vi "merge tdms files.vi"(0 "save to":path, 5 "merge paths":path[](array[path])) -> (14 "Dateipfad (Ausgang)":path, 19 "Fehler (Ausgang)":errorcluster)   [LabVIEW 2010, in "util.lvlib"]
uses:
  util.lvlib
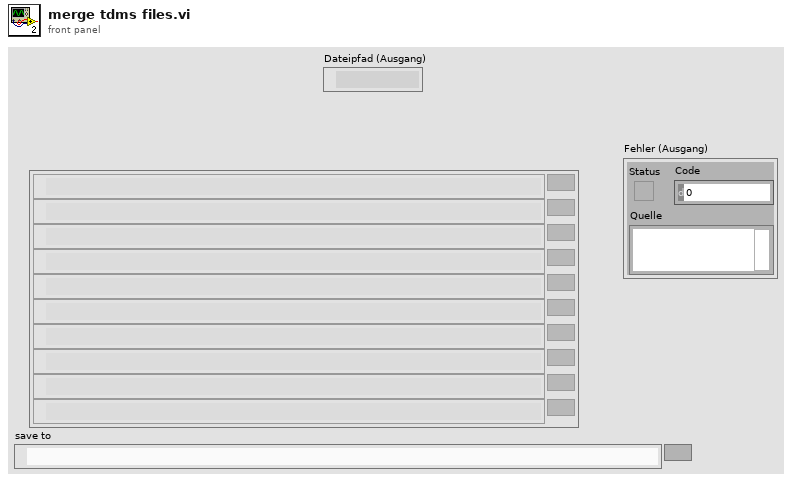
[diagram p1: front panel]
types:
  T1 = enum16{"open", "open or create", "create or replace", "create", "open (read-only)"}
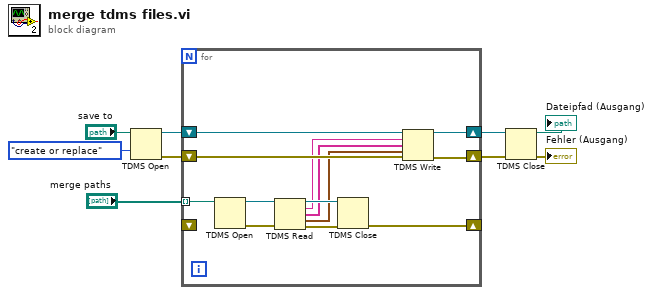
[diagram p0: block diagram]
diagram:
  n1 = TDMS Open(10:T1."create or replace" ("Operation (0:Öffnen)"), 11:"save to") -> (0:w8:errorcluster, 3:w9:refnum<k34>)  [unwired: 4 in]
  n2 = for {
    tunnel: "merge paths" -> [w22] mode=indexing
    shift-right: [w17] -> _
    shift-left: _ -> [_]
    shift-right: [w13] -> w7
    shift-left: w8 -> [w14]
    shift-right: [w15] -> w6
    shift-left: w9 -> [w16]
    n3 = TDMS Open(11:w22) -> (0:w19:errorcluster, 3:w21:refnum<k34>)  [unwired: 5 in]
    n4 = TDMS Read(0:w21, 11:w19) -> (4:w20:refnum<k34>, 6:w12:string, 8:w11:string[], 10:w10:waveform(dbl)[], 15:w18:errorcluster)  [unwired: 5 in, 1 out]
    n5 = TDMS Close(8:w18, 11:w20) -> (0:w17:errorcluster)  [unwired: 1 out]
    n6 = TDMS Write(0:w16, 5:w12, 7:w11, 9:w10, 11:w14) -> (4:w15:refnum<k34>, 15:w13:errorcluster)  [unwired: 1 in, 2 out]
  }
  n7 = TDMS Close(8:w7, 11:w6) -> (0:→"Fehler (Ausgang)":errorcluster, 3:→"Dateipfad (Ausgang)":path)
